vi "Format.vi"(6 "Statement":T1={"timestamp"=timestamp(0 s since 1904-01-01), "level"=enum."INFO", "sourceTag"="", "originVI"="", "message"=""}, 8 "error in (no error)":errorcluster, 11 "Layout in":refnum<class "Layout.lvclass">) -> (0 "error out":errorcluster, 3 "Layout out":refnum<class "Layout.lvclass">, 4 "FormattedLine":string)   [LabVIEW 2026, in "Lumberjack.lvlib" / "Layout.lvclass"]
doc: "Dynamic-dispatch, must-override. Convert one Statement into a single formatted output line (SRS-LMBR-015). The base defines the contract only; each concrete layout implements the formatting. Pure and stateless (no I/O, no actor context), so it is directly unit-testable."
uses:
  Layout.lvclass
  TypeDefs/Statement.ctl
  TypeDefs/Severity.ctl
  Lumberjack.lvlib
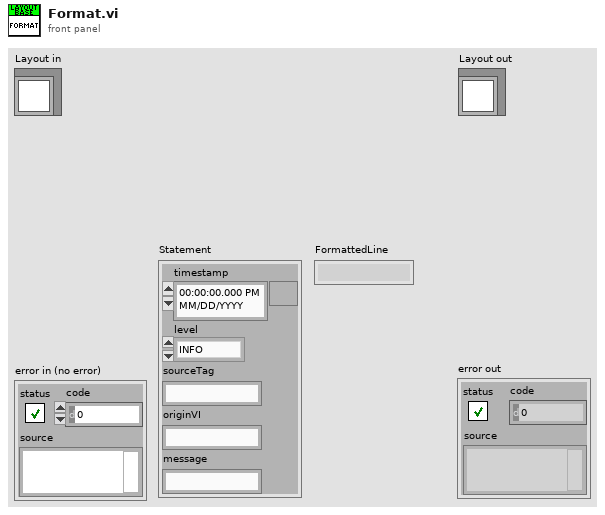
[diagram p1: front panel]
types:
  T1 = typedef "Lumberjack.lvlib/Statement.ctl" = cluster{"timestamp":timestamp, "level":T2, "sourceTag":string, "originVI":string, "message":string}
  T2 = typedef "Lumberjack.lvlib/Severity.ctl" = enum16{"OFF", "FATAL", "ERROR", "WARN", "INFO", "DEBUG", "TRACE", "ALL"}
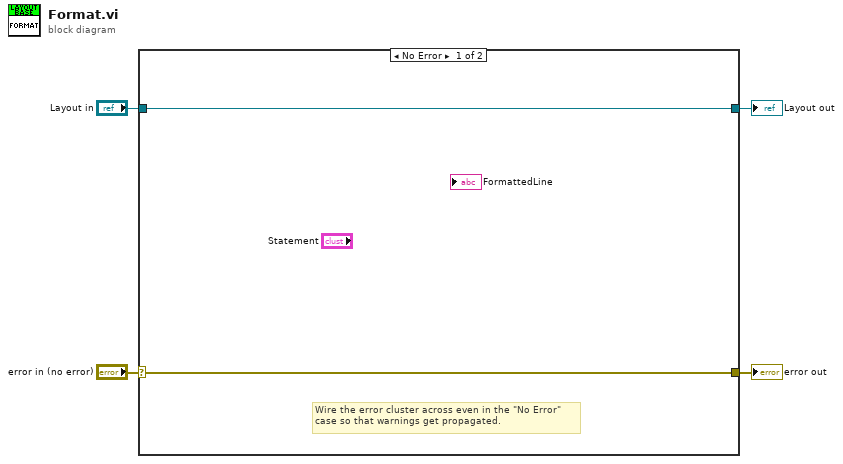
[diagram p0: block diagram]
diagram:
  n1 = case shown="No Error" "error in (no error)" {
    selector: "error in (no error)" -> [w6 w8]
    tunnel: [w6 w8] -> w3
    tunnel: [w5 w7] -> w1
    tunnel: "Layout in" -> [w5 w7]
    frame No Error {
      # "Wire the error cluster across even in the \"No Error\"\ncase so that warnings get propagated."
    }
    frame Error {
    }
  }
  "error out" <- w3
  "Layout out" <- w1
